vi "Fibonacci series.vi"() -> ()   [LabVIEW 2020]
panel:
  out "Array":i32[](array[numeric])
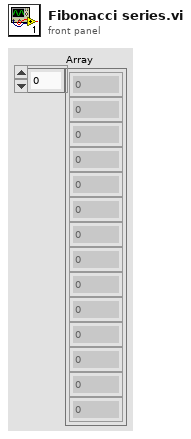
[diagram p1: front panel]
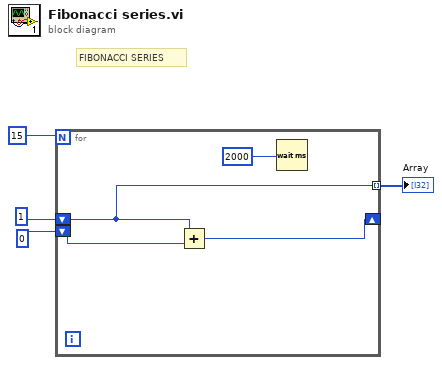
[diagram p0: block diagram]
diagram:
  # "FIBONACCI SERIES"
  n1 = for {
    N: 15 -> [_]
    shift-right: [w7] -> _
    shift-left: 0 -> [w8]
    shift-left: 1 -> [w6]
    tunnel: [w6] -> w2 mode=indexing
    n2 = Add(x=w6, y=w8) -> (x+y=w7:i32)
    n3 = Wait (ms)(milliseconds to wait=u32 2000) -> ()  [unwired: 1 out]
  }
  "Array" <- w2
